vi "Glueckwunsch(SubVI).vi"(0 "Array (Eingang)":refnum<vi>, 1 "Bool. Referenz":refnum<vi>, 2 "Game Over":bool, 5 "X Won":bool, 7 "Ring Referenz":refnum<vi>, 9 "O Won":bool, 12 "Str Referenz":refnum<vi>, 13 "reference":refnum<vi>, 14 "Arr Referenz (Eingang)":refnum<vi>) -> (4 "GewinnerRing":u16(ring)=1)   [LabVIEW 2017]
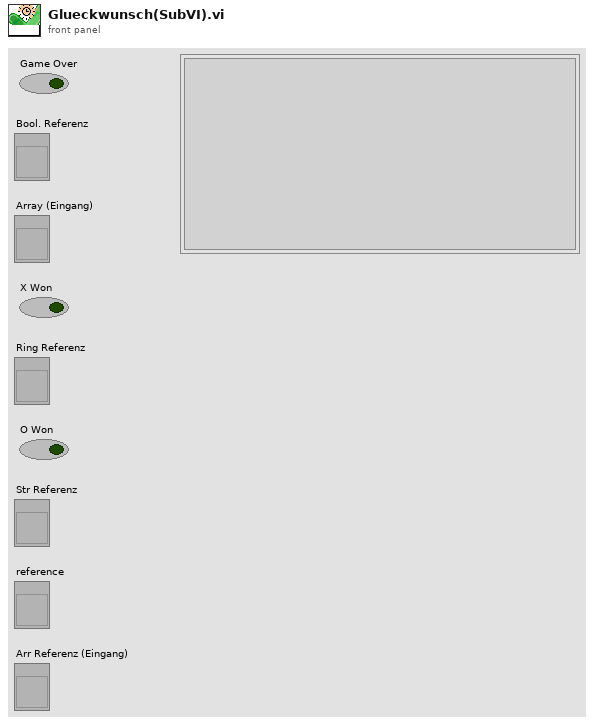
[diagram p1: front panel]
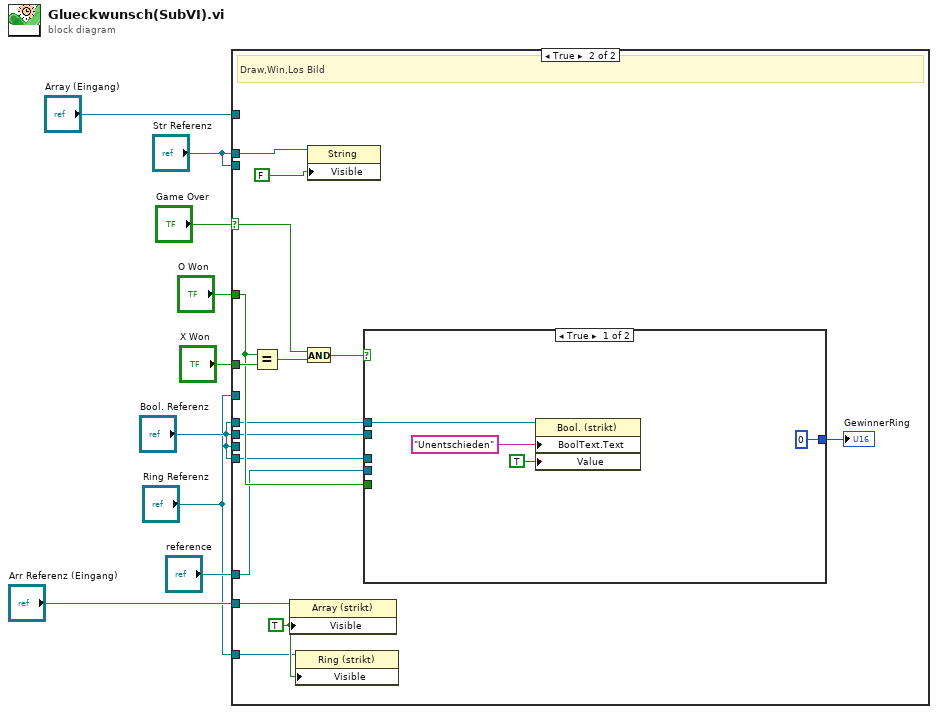
[diagram p0: block diagram]
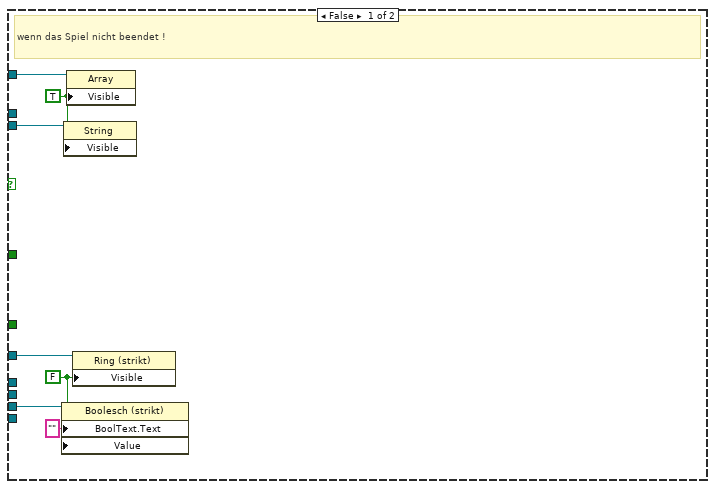
[diagram p2: hidden frame]
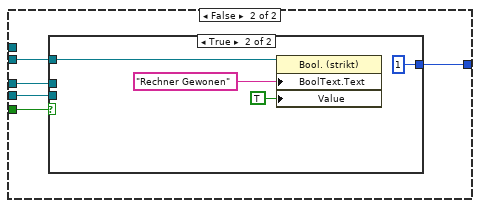
[diagram p3: hidden frame]
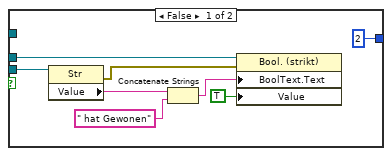
[diagram p4: hidden frame]
diagram:
  n1 = case shown="True" "Game Over" {
    selector: "Game Over" -> [_ w30]
    tunnel: "O Won" -> [_ w25]
    tunnel: "X Won" -> [_ w26]
    tunnel: "Array (Eingang)" -> [w13 _]
    tunnel: "Bool. Referenz" -> [w12 _]
    tunnel: "Ring Referenz" -> [w11 _]
    tunnel: "Str Referenz" -> [w10 _]
    tunnel: "Bool. Referenz" -> [_ w23]
    tunnel: "Bool. Referenz" -> [_ w22]
    tunnel: "reference" -> [_ w21]
    tunnel: "Bool. Referenz" -> [_ w20]
    tunnel: "Arr Referenz (Eingang)" -> [_ w19]
    tunnel: "Ring Referenz" -> [_ w18]
    tunnel: "Str Referenz" -> [_ w17]
    frame False {
      w15 = FALSE
      w14 = TRUE ("Sichtbar")
      # "wenn das Spiel nicht beendet !"
      n2 = property on="Eigenschaftsknoten" class="Boolesch (strikt)"(reference=w12, "BoolText.Text"="" ("Boolescher Text.Text"), "Value"=w15) -> ()  [unwired: 1 in, 2 out]
      n3 = property on="Eigenschaftsknoten" class="String"(reference=w10, "Visible"=w14) -> ()  [unwired: 1 in, 2 out]
      n4 = property on="Eigenschaftsknoten" class="Array"(reference=w13, "Visible"=w14) -> ()  [unwired: 1 in, 2 out]
      n5 = property on="Eigenschaftsknoten" class="Ring (strikt)"(reference=w11, "Visible"=w15) -> ()  [unwired: 1 in, 2 out]
    }
    frame True {
      w27 = TRUE ("Sichtbar")
      # "Draw,Win,Los Bild"
      n6 = Equal?(x=w25, y=w26) -> (x = y?=w24:bool)
      n7 = property on="Eigenschaftsknoten" class="Array (strikt)"(reference=w19, "Visible"=w27) -> ()  [unwired: 1 in, 2 out]
      n8 = property on="Eigenschaftsknoten" class="Ring (strikt)"(reference=w18, "Visible"=w27) -> ()  [unwired: 1 in, 2 out]
      n9 = And(x=w30, y=w24) -> (x .and. y?=w31:bool)
      n10 = property on="Eigenschaftsknoten" class="String"(reference=w17, "Visible"=FALSE) -> ()  [unwired: 1 in, 2 out]
      n11 = case shown="True" w31 {
        tunnel: w25 -> [_ w40]
        tunnel: [0 w39] -> w29
        tunnel: w23 -> [w32 _]
        tunnel: w22 -> [_ w38]
        tunnel: w21 -> [_ w37]
        tunnel: w20 -> [_ w36]
        frame True {
          n12 = property on="Eigenschaftsknoten" class="Bool. (strikt)"(reference=w32, "BoolText.Text"="Unentschieden" ("Boolescher Text.Text"), "Value"=TRUE) -> ()  [unwired: 1 in, 2 out]
        }
        frame False {
          n13 = case shown="True" w40 {
            tunnel: [2 1] -> w39
            tunnel: w38 -> [w43 _]
            tunnel: w37 -> [w42 _]
            tunnel: w36 -> [_ w49]
            frame False {
              n14 = property class="Str"(reference=w42) -> (error out=w41:errorcluster, "Value"=w47:string)  [unwired: 1 in, 1 out]
              n15 = Concatenate Strings(w47, " hat Gewonen" ("Boolescher Text.Text")) -> (w46:string)
              n16 = property on="Eigenschaftsknoten" class="Bool. (strikt)"(reference=w43, error in=w41, "BoolText.Text"=w46, "Value"=TRUE) -> ()  [unwired: 2 out]
            }
            frame True {
              n17 = property on="Eigenschaftsknoten" class="Bool. (strikt)"(reference=w49, "BoolText.Text"="Rechner Gewonen" ("Boolescher Text.Text"), "Value"=TRUE) -> ()  [unwired: 1 in, 2 out]
            }
          }
        }
      }
      "GewinnerRing" <- w29
    }
  }
